vi "Instrument Sequence Loop.vi"(6 "Which Program?":T1, 8 "error in":errorcluster, 10 "Message Queues out":T15, 11 "Notifiers":T2) -> (0 "error out":errorcluster)   [LabVIEW 2014]
uses:
  support/Message Queue/All Message Queues.ctl
  support/Message Queue/Message Cluster.ctl
  support/Notifiers/Notifiers.ctl
  support/Message Handler Loop Notifiers.ctl
  Hardware Control/Parameter Analyzer/Parameter Analyzer Notifiers.ctl
  Hardware Control/Switching Matrix/Switching Matrix Notifiers.ctl
  Hardware Control/Stress Control/StressControl Notifiers.ctl
  Hardware Control/Spectrometer/Spectrometer Notifiers.ctl
  Hardware Control/Switches and Mirrors/SwitchesMirrors Notifiers.ctl
  Hardware Control/Camera/Camera Notifiers.ctl
  Hardware Control/XYZ Stage/XYZ Notifications.ctl
  Hardware Control/Autofocus/Autofocus Notifiers.ctl
  Measurements/Optoelectronic Measurement/Optoelectronic Notifiers.ctl
  Measurements/Save Data/SaveData Notifiers.ctl
  Measurements/Instrument Sequence/Instrument Sequence Notifiers.ctl
  Measurements/Instrument Sequence/Instrument Stequence - Which Program.ctl
  Measurements/Instrument Sequence/Instrument Sequence Function.ctl
  support/Message Queue/Message Queue.lvlib
panel:
  # "LICENSED MATERIALS – PROPERTY OF IBM\nCopyright IBM Corp. 2016,\nALL RIGHTS RESERVED"
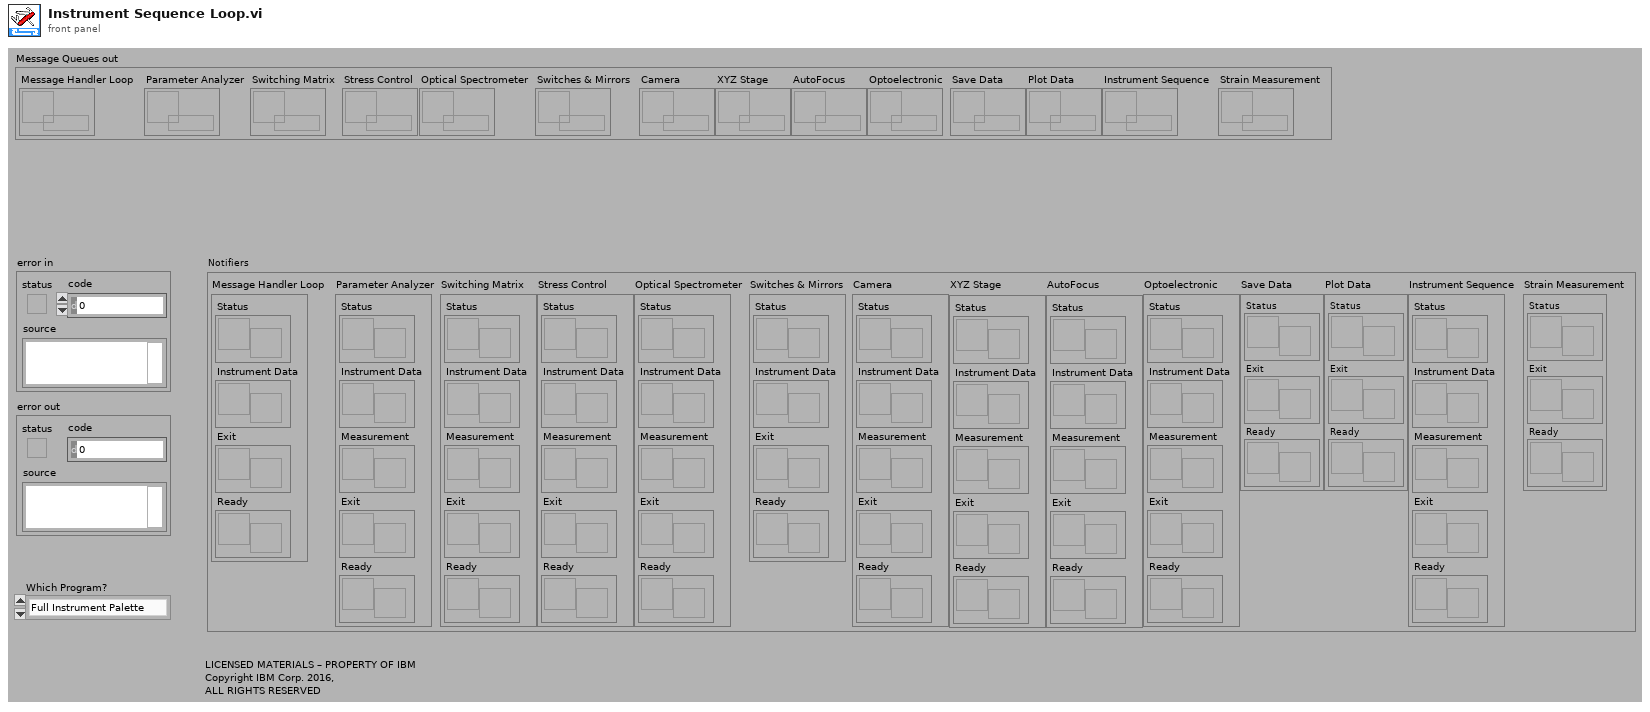
[diagram p1: front panel]
types:
  T1 = typedef "Instrument Stequence - Which Program.ctl" = enum16{"Full Instrument Palette", "Strain Electrical"}
  T2 = typedef "Notifiers.ctl" = cluster{"Message Handler Loop":T3, "Parameter Analyzer":T4, "Switching Matrix":T5, "Stress Control":T6, "Optical Spectrometer":T7, "Switches & Mirrors":T8, "Camera":T9, "XYZ Stage":T10, "AutoFocus":T11, "Optoelectronic":T12, "Save Data":T13, "Plot Data":T13, "Instrument Sequence":T14, "Strain Measurement":cluster{"Status":refnum<notifier>, "Exit":refnum<notifier>, "Ready":refnum<notifier>}}
  T3 = typedef "Message Handler Loop Notifiers.ctl" = cluster{"Status":refnum<notifier>, "Instrument Data":refnum<notifier>, "Exit":refnum<notifier>, "Ready":refnum<notifier>}
  T4 = typedef "Parameter Analyzer Notifiers.ctl" = cluster{"Status":refnum<notifier>, "Instrument Data":refnum<notifier>, "Measurement":refnum<notifier>, "Exit":refnum<notifier>, "Ready":refnum<notifier>}
  T5 = typedef "Switching Matrix Notifiers.ctl" = cluster{"Status":refnum<notifier>, "Instrument Data":refnum<notifier>, "Measurement":refnum<notifier>, "Exit":refnum<notifier>, "Ready":refnum<notifier>}
  T6 = typedef "StressControl Notifiers.ctl" = cluster{"Status":refnum<notifier>, "Instrument Data":refnum<notifier>, "Measurement":refnum<notifier>, "Exit":refnum<notifier>, "Ready":refnum<notifier>}
  T7 = typedef "Spectrometer Notifiers.ctl" = cluster{"Status":refnum<notifier>, "Instrument Data":refnum<notifier>, "Measurement":refnum<notifier>, "Exit":refnum<notifier>, "Ready":refnum<notifier>}
  T8 = typedef "SwitchesMirrors Notifiers.ctl" = cluster{"Status":refnum<notifier>, "Instrument Data":refnum<notifier>, "Exit":refnum<notifier>, "Ready":refnum<notifier>}
  T9 = typedef "Camera Notifiers.ctl" = cluster{"Status":refnum<notifier>, "Instrument Data":refnum<notifier>, "Measurement":refnum<notifier>, "Exit":refnum<notifier>, "Ready":refnum<notifier>}
  T10 = typedef "XYZ Notifications.ctl" = cluster{"Status":refnum<notifier>, "Instrument Data":refnum<notifier>, "Measurement":refnum<notifier>, "Exit":refnum<notifier>, "Ready":refnum<notifier>}
  T11 = typedef "Autofocus Notifiers.ctl" = cluster{"Status":refnum<notifier>, "Instrument Data":refnum<notifier>, "Measurement":refnum<notifier>, "Exit":refnum<notifier>, "Ready":refnum<notifier>}
  T12 = typedef "Optoelectronic Notifiers.ctl" = cluster{"Status":refnum<notifier>, "Instrument Data":refnum<notifier>, "Measurement":refnum<notifier>, "Exit":refnum<notifier>, "Ready":refnum<notifier>}
  T13 = typedef "SaveData Notifiers.ctl" = cluster{"Status":refnum<notifier>, "Exit":refnum<notifier>, "Ready":refnum<notifier>}
  T14 = typedef "Instrument Sequence Notifiers.ctl" = cluster{"Status":refnum<notifier>, "Instrument Data":refnum<notifier>, "Measurement":refnum<notifier>, "Exit":refnum<notifier>, "Ready":refnum<notifier>}
  T15 = typedef "Message Queue.lvlib/All Message Queues.ctl" = cluster{"Message Handler Loop":refnum<queue>, "Parameter Analyzer":refnum<queue>, "Switching Matrix":refnum<queue>, "Stress Control":refnum<queue>, "Optical Spectrometer":refnum<queue>, "Switches & Mirrors":refnum<queue>, "Camera":refnum<queue>, "XYZ Stage":refnum<queue>, "AutoFocus":refnum<queue>, "Optoelectronic":refnum<queue>, "Save Data":refnum<queue>, "Plot Data":refnum<queue>, "Instrument Sequence":refnum<queue>, "Strain Measurement":refnum<queue>}
  T16 = typedef "Instrument Sequence Data.ctl" = cluster{"Configuration":T17, "Refnums":T18}
  T17 = typedef "Instrument Sequence Config.ctl" = cluster{"Caller VI":enum16{"User", "Stress Measurement VI"}}
  T18 = typedef "Instrument Sequence Refnums.ctl" = cluster{"Instrument Steps":refnum<vi>, "Instruments Status":refnum<vi>, "Device ID":refnum<vi>, "Device Information":refnum<vi>, "Pause-Resume":refnum<vi>, "Plot":T19}
  T19 = typedef "Electrical Data Plot Refnums.ctl" = cluster{"Plot List":refnum<vi>, "Voltage Plot":refnum<vi>, "Current Plot":refnum<vi>, "IV Characteristic":refnum<vi>, "dI/dV-V Characteristic":refnum<vi>}
  T20 = typedef "Instrument Sequence Function.ctl" = enum16{"Update Refnums", "Get Instruments Status", "Initialize Dialog", "Get Autofocus Status", "Add Step", "Remove Step", "Clear Sequence", "Load Sequence", "Save Sequence", "Measure Sequence", "Reset Sequence", "Start Sequence", "Start Sequence for Strain Measurement", "Stop Sequence", "Pause Sequence", "Update Sequence Status", "Choose What Next", "Update Workspace Data", "Save Measured Sequence", "Configure Parameter Analyzer", "Perform Electrical Measurement", "Configure Switching Matrix", "Configure Optical Spectrometer", "Focus", "Perform Optical Measurement", "Perform Optoelectronic Measurement", "Declare Completion"}
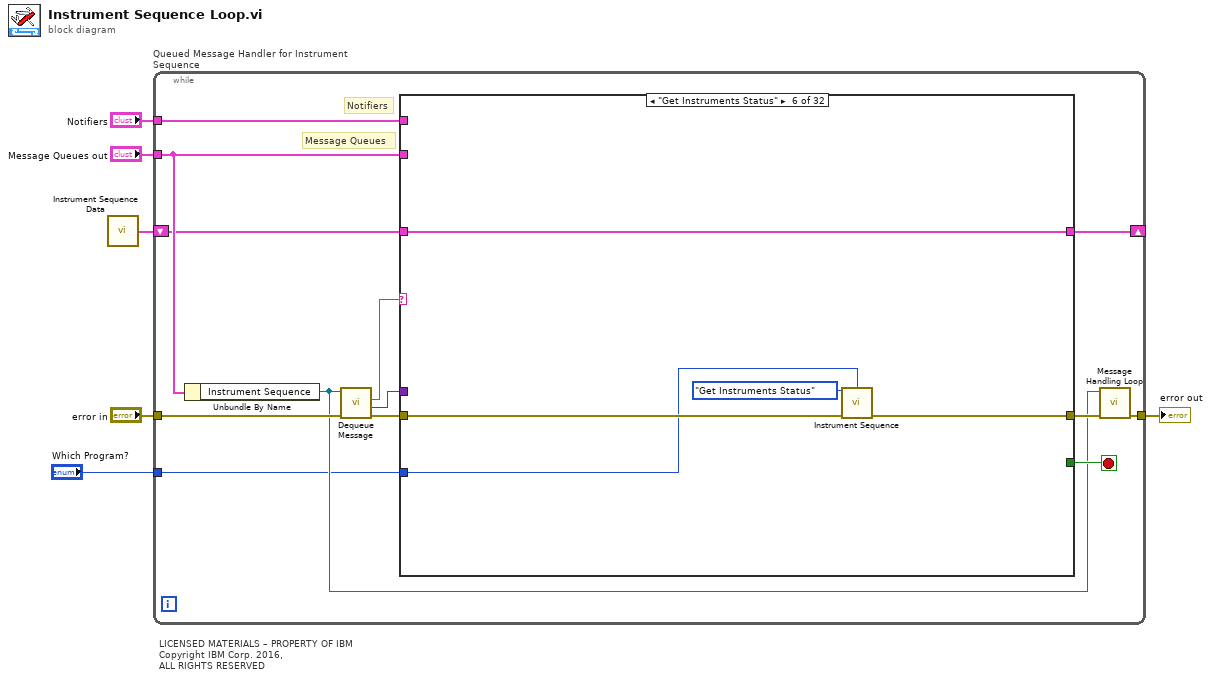
[diagram p0: block diagram]
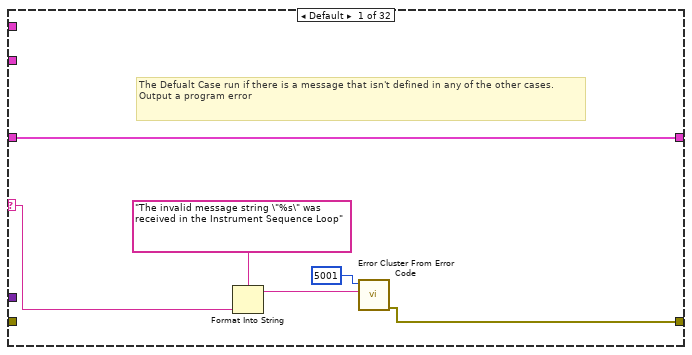
[diagram p2: hidden frame]
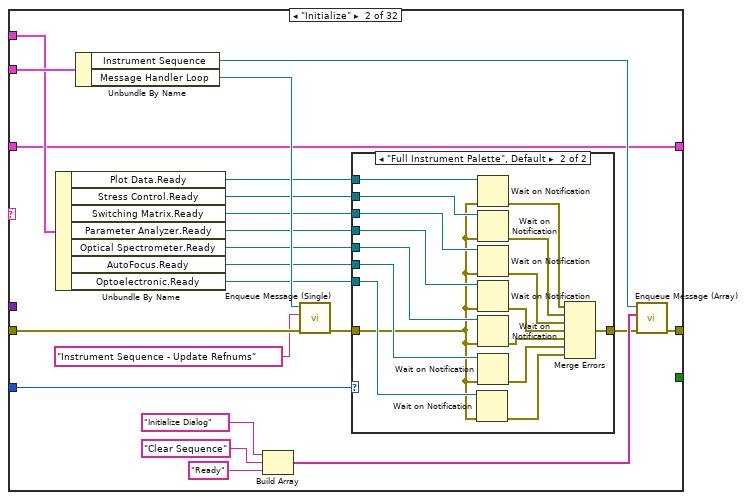
[diagram p3: hidden frame]
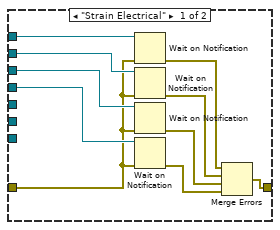
[diagram p4: hidden frame]
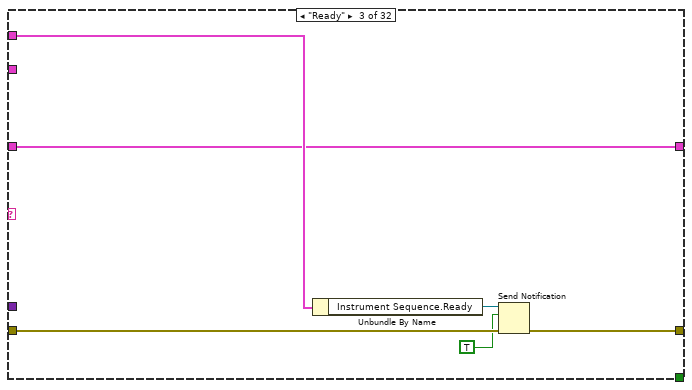
[diagram p5: hidden frame]
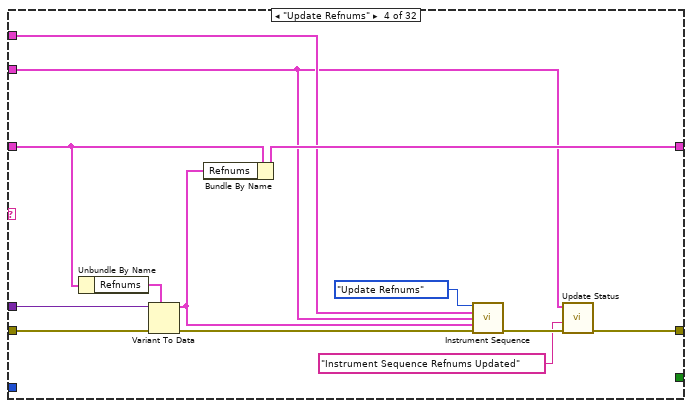
[diagram p6: hidden frame]
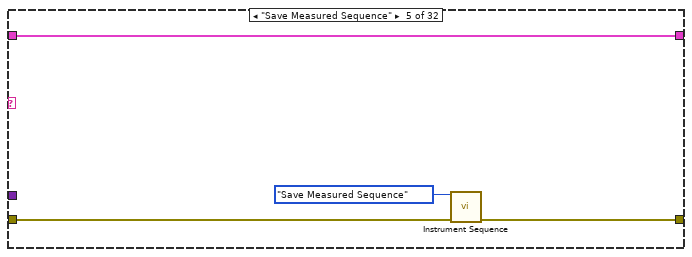
[diagram p7: hidden frame]
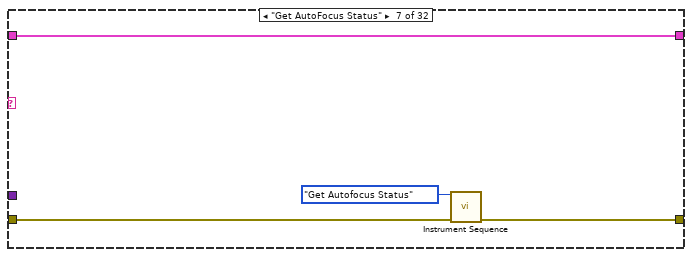
[diagram p8: hidden frame]
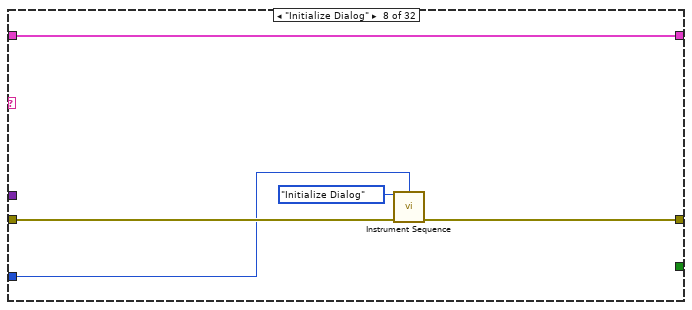
[diagram p9: hidden frame]
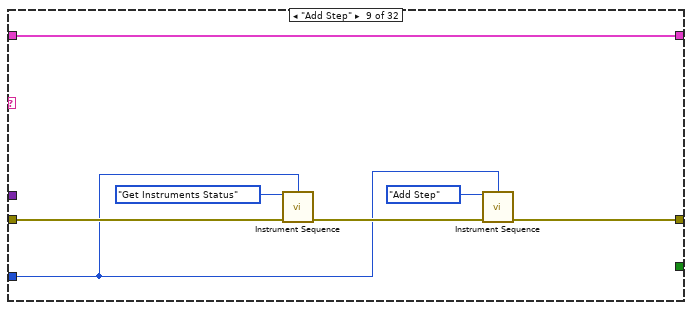
[diagram p10: hidden frame]
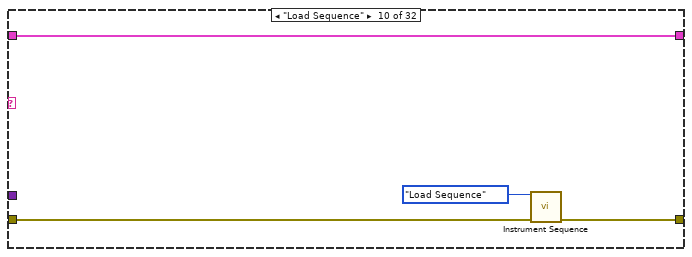
[diagram p11: hidden frame]
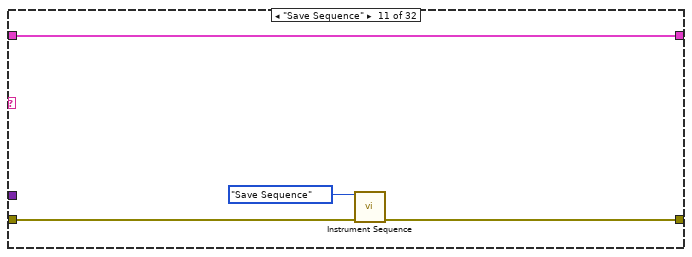
[diagram p12: hidden frame]
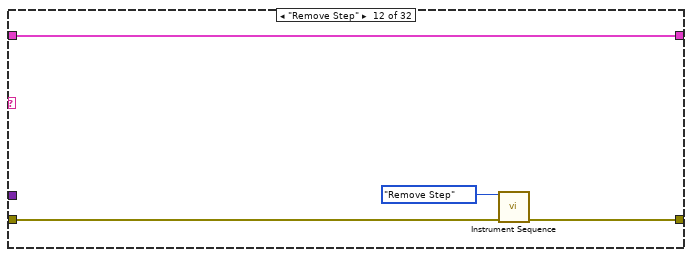
[diagram p13: hidden frame]
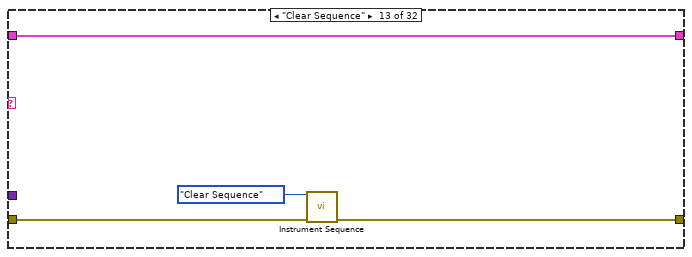
[diagram p14: hidden frame]
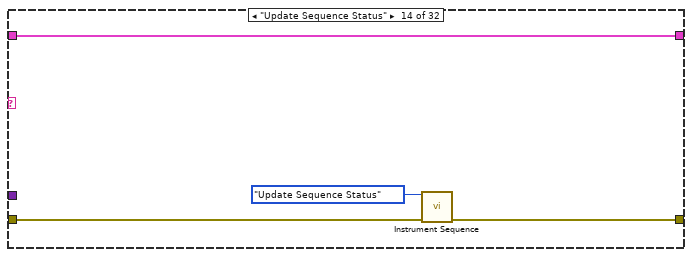
[diagram p15: hidden frame]
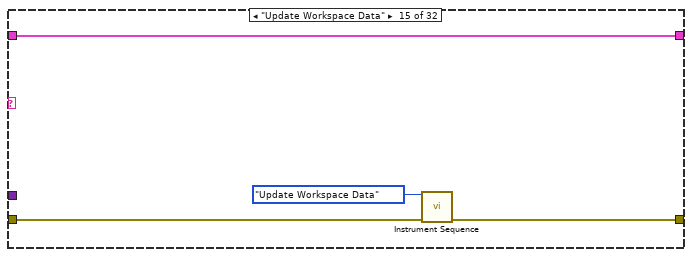
[diagram p16: hidden frame]
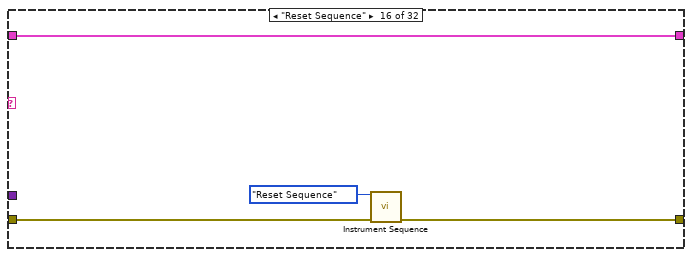
[diagram p17: hidden frame]
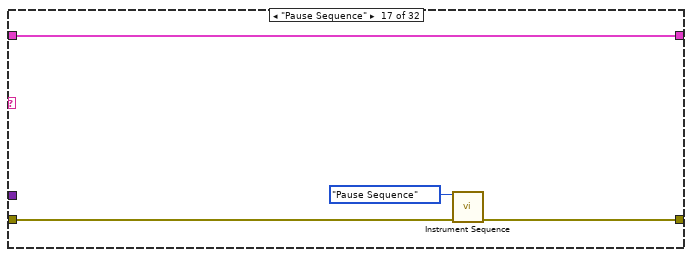
[diagram p18: hidden frame]
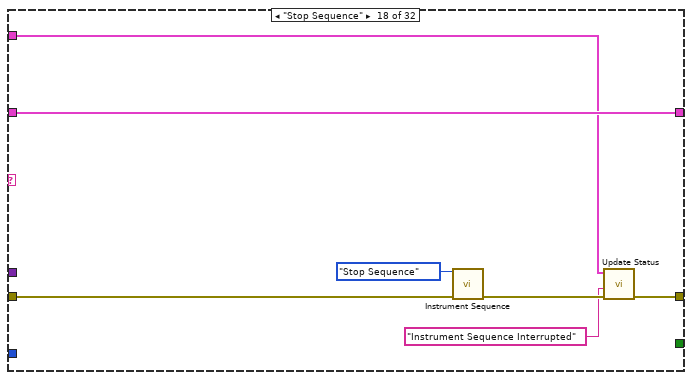
[diagram p19: hidden frame]
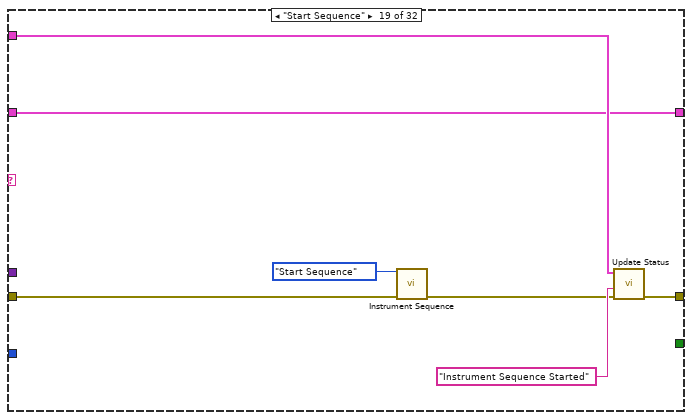
[diagram p20: hidden frame]
diagram:
  # "LICENSED MATERIALS – PROPERTY OF IBM\nCopyright IBM Corp. 2016,\nALL RIGHTS RESERVED"
  n1 = call "Instrument Sequence Data.vi"() -> ("Instrument Sequence Data"=w2:T16)
  n2 = while "Queued Message Handler for Instrument Sequence" {
    tunnel: "error in" -> [w19]
    tunnel: [w11] -> w3
    tunnel: "Message Queues out" -> [w15]
    tunnel: "Notifiers" -> [w14]
    shift-right: [w8] -> _
    shift-left: w2 -> [w9]
    tunnel: "Which Program?" -> [w7]
    stop <- w13 stop-if-true
    # "Notifiers"
    # "Message Queues"
    n3 = Unbundle By Name(w15) -> ("Instrument Sequence"=w10:refnum<queue>)
    n4 = call "Dequeue Message.vi"("error in (no error)"=w19, "Message Queue"=w10) -> ("error out"=w18:errorcluster, "Message Data"=w16:variant, "Message"=w17:string)  [unwired: 7 out]
    n5 = case shown="\"Get Instruments Status\"" w17 {
      selector: w17 -> [w22 _ _ _ _ _ _ _ _ _ _ _ _ _ _ _ _ _ _ _ _ _ _ _ _ _ _ _ _ _ _ _]
      tunnel: w18 -> [_ w45 w76 w91 w95 w99 w103 w109 w113 w118 w122 w126 w131 w136 w140 w142 w147 w154 w158 w169 w175 w182 w190 w199 w205 w210 w214 w217 w221 w225 w236 w251]
      tunnel: [w21 w37 w79 w90 w93 w98 w102 w108 w115 w119 w124 w127 w130 w134 w138 w144 w146 w152 w162 w170 w173 w183 w188 w201 w204 w209 w213 w216 w220 w224 w231 w244] -> w12
      tunnel: w16 -> [_ _ _ w92 _ _ _ _ _ _ _ _ _ _ _ _ _ _ _ w167 _ w179 _ w197 w202 w207 _ _ _ _ w229 _]
      tunnel: w15 -> [_ w47 _ w84 _ _ _ _ _ _ _ _ _ _ _ _ _ w151 w161 _ _ _ w186 _ _ _ _ _ _ _ w237 w254]
      tunnel: w14 -> [_ w46 w77 w85 _ _ _ _ _ _ _ _ _ _ _ _ _ _ _ _ _ _ _ _ _ _ _ _ _ _ _ w246]
      tunnel: [_ _ _ _ _ _ _ _ _ _ _ _ _ _ _ _ _ _ _ _ _ _ _ _ _ _ _ _ _ _ _ TRUE ("Priority Message? (F)")] -> w13
      tunnel: w9 -> [w20 w33 w74 w88 w96 w101 w105 w110 w116 w120 w123 w128 w132 w137 w141 w143 w149 w156 w159 w166 w174 w181 w189 w198 w206 w211 w215 w219 w223 w227 w228 w252]
      tunnel: [w20 w33 w74 w89 w96 w101 w105 w110 w116 w120 w123 w128 w132 w137 w141 w143 w149 w156 w159 w171 w174 w178 w189 w198 w206 w211 w215 w219 w223 w227 w228 w252] -> w8
      tunnel: w7 -> [_ w27 _ _ _ w97 _ w106 w111 _ _ _ _ _ _ _ _ _ _ _ _ _ _ _ _ _ _ _ _ _ _ _]
      frame Default {
        # "The Defualt Case run if there is a message that isn't defined in any of the other cases.\nOutput a program error"
        n6 = Format Into String(format string="The invalid message string \"%s\" was  received in the Instrument Sequence Loop", w22) -> (resulting string=w24:string)  [unwired: 2 in, 1 out]
        n7 = call <vilib>:"Error Cluster From Error Code.vi"("error message (\"\")"=w24, "error code (0)"=5001) -> ("error out"=w21:errorcluster)  [unwired: 2 in, 5 out]
      }
      frame "Initialize" {
        n8 = Unbundle By Name(w46) -> ("Plot Data.Ready"=w28:refnum<notifier>, "Stress Control.Ready"=w40:refnum<notifier>, "Switching Matrix.Ready"=w42:refnum<notifier>, "Parameter Analyzer.Ready"=w41:refnum<notifier>, "Optical Spectrometer.Ready"=w31:refnum<notifier>, "AutoFocus.Ready"=w30:refnum<notifier>, "Optoelectronic.Ready"=w26:refnum<notifier>)
        n9 = Unbundle By Name(w47) -> ("Instrument Sequence"=w39:refnum<queue>, "Message Handler Loop"=w43:refnum<queue>)
        n10 = Build Array("Initialize Dialog" ("Message"), "Clear Sequence" ("Message"), "Ready" ("Message")) -> (w38:string[])
        n11 = call "Enqueue Message (Single).vi"("error in (no error)"=w45, "Message"="Instrument Sequence - Update Refnums", "Message Queue"=w43) -> ("error out"=w29:errorcluster)  [unwired: 1 in, 7 out]
        n12 = case shown="\"Full Instrument Palette\", Default" w27 {
          tunnel: w42 -> [w57 w73]
          tunnel: w41 -> [w56 w72]
          tunnel: w40 -> [w54 w70]
          tunnel: [w50 w66] -> w32
          tunnel: w31 -> [_ w64]
          tunnel: w30 -> [_ w63]
          tunnel: w29 -> [w49 w59]
          tunnel: w28 -> [w48 w61]
          tunnel: w26 -> [_ w60]
          frame "Strain Electrical" {
            n13 = Wait on Notification(notifier=w48, error in (no error)=w49) -> (error out=w51:errorcluster)  [unwired: 5 out]
            n14 = Wait on Notification(notifier=w54, error in (no error)=w49) -> (error out=w52:errorcluster)  [unwired: 5 out]
            n15 = Wait on Notification(notifier=w57, error in (no error)=w49) -> (error out=w53:errorcluster)  [unwired: 5 out]
            n16 = Wait on Notification(notifier=w56, error in (no error)=w49) -> (error out=w55:errorcluster)  [unwired: 5 out]
            n17 = Merge Errors(w51, w52, w53, w55) -> (w50:errorcluster)
          }
          frame "Full Instrument Palette", Default {
            n18 = Wait on Notification(notifier=w60, error in (no error)=w59) -> (error out=w58:errorcluster)  [unwired: 5 out]
            n19 = Wait on Notification(notifier=w61, error in (no error)=w59) -> (error out=w67:errorcluster)  [unwired: 5 out]
            n20 = Wait on Notification(notifier=w70, error in (no error)=w59) -> (error out=w68:errorcluster)  [unwired: 5 out]
            n21 = Wait on Notification(notifier=w73, error in (no error)=w59) -> (error out=w69:errorcluster)  [unwired: 5 out]
            n22 = Wait on Notification(notifier=w72, error in (no error)=w59) -> (error out=w71:errorcluster)  [unwired: 5 out]
            n23 = Wait on Notification(notifier=w64, error in (no error)=w59) -> (error out=w65:errorcluster)  [unwired: 5 out]
            n24 = Wait on Notification(notifier=w63, error in (no error)=w59) -> (error out=w62:errorcluster)  [unwired: 5 out]
            n25 = Merge Errors(w67, w68, w69, w71, w65, w62, w58) -> (w66:errorcluster)
          }
        }
        n26 = call "Enqueue Message (Array).vi"("error in (no error)"=w32, "Message Array"=w38, "Message Queue"=w39) -> ("error out"=w37:errorcluster)  [unwired: 1 in, 7 out]
      }
      frame "Ready" {
        n27 = Unbundle By Name(w77) -> ("Instrument Sequence.Ready"=w78:refnum<notifier>)
        n28 = Send Notification(notification=TRUE, notifier=w78, error in (no error)=w76) -> (error out=w79:errorcluster)  [unwired: 1 out]
      }
      frame "Update Refnums" {
        n29 = Unbundle By Name(w88) -> ("Refnums"=w87:T18)
        n30 = Variant To Data(error in=w91, type=w87, Variant=w92) -> (data=w81:T18, error out=w83:errorcluster)
        n31 = Bundle By Name(cluster=w88, "Refnums"=w81) -> (w89:T16)
        n32 = call "Instrument Sequence.vi"("Function"=Instrument_Sequence_Function."Update Refnums", "Notifiers"=w85, "Message Queues"=w84, "Refnums"=w81, "error in (no error)"=w83) -> ("error out"=w82:errorcluster)  [unwired: 3 in, 7 out]
        n33 = call "Update Status.vi"("error in"=w82, "String"="Instrument Sequence Refnums Updated", "Message Queues out"=w84) -> ("error out"=w90:errorcluster)  [unwired: 8 out]
      }
      frame "Save Measured Sequence" {
        n34 = call "Instrument Sequence.vi"("Function"=Instrument_Sequence_Function."Save Measured Sequence", "error in (no error)"=w95) -> ("error out"=w93:errorcluster)  [unwired: 6 in, 7 out]
      }
      frame "Get Instruments Status" {
        n35 = call "Instrument Sequence.vi"("Function"=Instrument_Sequence_Function."Get Instruments Status", "Which Program?"=w97, "error in (no error)"=w99) -> ("error out"=w98:errorcluster)  [unwired: 5 in, 7 out]
      }
      frame "Get AutoFocus Status" {
        n36 = call "Instrument Sequence.vi"("Function"=Instrument_Sequence_Function."Get Autofocus Status", "error in (no error)"=w103) -> ("error out"=w102:errorcluster)  [unwired: 6 in, 7 out]
      }
      frame "Initialize Dialog" {
        n37 = call "Instrument Sequence.vi"("Function"=Instrument_Sequence_Function."Initialize Dialog", "Which Program?"=w106, "error in (no error)"=w109) -> ("error out"=w108:errorcluster)  [unwired: 5 in, 7 out]
      }
      frame "Add Step" {
        n38 = call "Instrument Sequence.vi"("Function"=Instrument_Sequence_Function."Get Instruments Status", "Which Program?"=w111, "error in (no error)"=w113) -> ("error out"=w112:errorcluster)  [unwired: 5 in, 7 out]
        n39 = call "Instrument Sequence.vi"("Function"=Instrument_Sequence_Function."Add Step", "Which Program?"=w111, "error in (no error)"=w112) -> ("error out"=w115:errorcluster)  [unwired: 5 in, 7 out]
      }
      frame "Load Sequence" {
        n40 = call "Instrument Sequence.vi"("Function"=Instrument_Sequence_Function."Load Sequence", "error in (no error)"=w118) -> ("error out"=w119:errorcluster)  [unwired: 6 in, 7 out]
      }
      frame "Save Sequence" {
        n41 = call "Instrument Sequence.vi"("Function"=Instrument_Sequence_Function."Save Sequence", "error in (no error)"=w122) -> ("error out"=w124:errorcluster)  [unwired: 6 in, 7 out]
      }
      frame "Remove Step" {
        n42 = call "Instrument Sequence.vi"("Function"=Instrument_Sequence_Function."Remove Step", "error in (no error)"=w126) -> ("error out"=w127:errorcluster)  [unwired: 6 in, 7 out]
      }
      frame "Clear Sequence" {
        n43 = call "Instrument Sequence.vi"("Function"=Instrument_Sequence_Function."Clear Sequence", "error in (no error)"=w131) -> ("error out"=w130:errorcluster)  [unwired: 6 in, 7 out]
      }
      frame "Update Sequence Status" {
        n44 = call "Instrument Sequence.vi"("Function"=Instrument_Sequence_Function."Update Sequence Status", "error in (no error)"=w136) -> ("error out"=w134:errorcluster)  [unwired: 6 in, 7 out]
      }
      frame "Update Workspace Data" {
        n45 = call "Instrument Sequence.vi"("Function"=Instrument_Sequence_Function."Update Workspace Data", "error in (no error)"=w140) -> ("error out"=w138:errorcluster)  [unwired: 6 in, 7 out]
      }
      frame "Reset Sequence" {
        n46 = call "Instrument Sequence.vi"("Function"=Instrument_Sequence_Function."Reset Sequence", "error in (no error)"=w142) -> ("error out"=w144:errorcluster)  [unwired: 6 in, 7 out]
      }
      frame "Pause Sequence" {
        n47 = call "Instrument Sequence.vi"("Function"=Instrument_Sequence_Function."Pause Sequence", "error in (no error)"=w147) -> ("error out"=w146:errorcluster)  [unwired: 6 in, 7 out]
      }
      frame "Stop Sequence" {
        n48 = call "Instrument Sequence.vi"("Function"=Instrument_Sequence_Function."Stop Sequence", "error in (no error)"=w154) -> ("error out"=w153:errorcluster)  [unwired: 6 in, 7 out]
        n49 = call "Update Status.vi"("error in"=w153, "String"="Instrument Sequence Interrupted", "Message Queues out"=w151) -> ("error out"=w152:errorcluster)  [unwired: 8 out]
      }
      frame "Start Sequence" {
        n50 = call "Instrument Sequence.vi"("Function"=Instrument_Sequence_Function."Start Sequence", "error in (no error)"=w158) -> ("error out"=w157:errorcluster)  [unwired: 6 in, 7 out]
        n51 = call "Update Status.vi"("error in"=w157, "String"="Instrument Sequence Started", "Message Queues out"=w161) -> ("error out"=w162:errorcluster)  [unwired: 8 out]
      }
      frame "Measure Sequence" {
        n52 = Unbundle By Name(w166) -> ("Configuration.Caller VI"=w165:enum16{"User", "Stress Measurement VI"})
        n53 = Variant To Data(error in=w169, type=w165, Variant=w167) -> (data=w164:enum16{"User", "Stress Measurement VI"}, error out=w168:errorcluster)
        n54 = call "Instrument Sequence.vi"("Function"=Instrument_Sequence_Function."Measure Sequence", "Caller VI"=w164, "error in (no error)"=w168) -> ("error out"=w170:errorcluster)  [unwired: 5 in, 7 out]
        n55 = Bundle By Name(cluster=w166, "Configuration.Caller VI"=w164) -> (w171:T16)
      }
      frame "Start Sequence for Strain Measurement" {
        n56 = call "Instrument Sequence.vi"("Function"=Instrument_Sequence_Function."Start Sequence for Strain Measurement", "error in (no error)"=w175) -> ("error out"=w173:errorcluster)  [unwired: 6 in, 7 out]
      }
      frame "Choose What Next" {
        n57 = Unbundle By Name(w181) -> ("Configuration.Caller VI"=w177:enum16{"User", "Stress Measurement VI"})
        n58 = Variant To Data(error in=w182, type=w177, Variant=w179) -> (error out=w180:errorcluster)  [unwired: 1 out]
        n59 = call "Instrument Sequence.vi"("Function"=Instrument_Sequence_Function."Choose What Next", "Caller VI"=w177, "error in (no error)"=w180) -> ("error out"=w183:errorcluster)  [unwired: 5 in, 7 out]
        n60 = Bundle By Name(cluster=w181, "Configuration.Caller VI"=w177) -> (w178:T16)
      }
      frame "Declare Completion" {
        n61 = Unbundle By Name(w189) -> ("Configuration.Caller VI"=w185:enum16{"User", "Stress Measurement VI"})
        n62 = call "Instrument Sequence.vi"("Function"=Instrument_Sequence_Function."Declare Completion", "Caller VI"=w185, "error in (no error)"=w190) -> ("error out"=w187:errorcluster)  [unwired: 5 in, 7 out]
        n63 = case shown="\"User\", Default" w185 {
          tunnel: [w195 w196] -> w188
          tunnel: w187 -> [w194 w196]
          tunnel: w186 -> [w193 _]
          frame "User", Default {
            n64 = call "Update Status.vi"("error in"=w194, "String"="Instrument Sequence Completed", "Message Queues out"=w193) -> ("error out"=w195:errorcluster)  [unwired: 8 out]
          }
          frame "Stress Measurement VI" {
          }
        }
      }
      frame "Configure Parameter Analyzer" {
        n65 = call "Instrument Sequence.vi"("Function"=Instrument_Sequence_Function."Configure Parameter Analyzer", "error in (no error)"=w199, "Configuration"=w197) -> ("error out"=w201:errorcluster)  [unwired: 5 in, 7 out]
      }
      frame "Configure Switching Matrix" {
        n66 = call "Instrument Sequence.vi"("Function"=Instrument_Sequence_Function."Configure Switching Matrix", "error in (no error)"=w205, "Configuration"=w202) -> ("error out"=w204:errorcluster)  [unwired: 5 in, 7 out]
      }
      frame "Configure Optical Spectrometer" {
        n67 = call "Instrument Sequence.vi"("Function"=Instrument_Sequence_Function."Configure Optical Spectrometer", "error in (no error)"=w210, "Configuration"=w207) -> ("error out"=w209:errorcluster)  [unwired: 5 in, 7 out]
      }
      frame "Focus" {
        n68 = call "Instrument Sequence.vi"("Function"=Instrument_Sequence_Function."Focus", "error in (no error)"=w214) -> ("error out"=w213:errorcluster)  [unwired: 6 in, 7 out]
      }
      frame "Perform Electrical Measurement" {
        n69 = call "Instrument Sequence.vi"("Function"=Instrument_Sequence_Function."Perform Electrical Measurement", "error in (no error)"=w217) -> ("error out"=w216:errorcluster)  [unwired: 6 in, 7 out]
      }
      frame "Perform Optical Measurement" {
        n70 = call "Instrument Sequence.vi"("Function"=Instrument_Sequence_Function."Perform Optical Measurement", "error in (no error)"=w221) -> ("error out"=w220:errorcluster)  [unwired: 6 in, 7 out]
      }
      frame "Perform Optoelectronic Measurement" {
        n71 = call "Instrument Sequence.vi"("Function"=Instrument_Sequence_Function."Perform Optoelectronic Measurement", "error in (no error)"=w225) -> ("error out"=w224:errorcluster)  [unwired: 6 in, 7 out]
      }
      frame "Error" {
        # "Clear Errors to avoid getting stuck \nin repeating this case"
        # "Add here Cases that are handled \nalready by the Message Handler Loop"
        n72 = Variant To Data(error in=w236, type=errorcluster {"status"=FALSE, "code"=0, "source"=""} ("error out"), Variant=w229) -> (data=w235:errorcluster, error out=w234:errorcluster)
        n73 = Merge Errors(w235, w234) -> (w233:errorcluster)
        n74 = Unbundle By Name(w237) -> ("Message Handler Loop"=w239:refnum<queue>)
        n75 = Unbundle By Name(w233) -> ("code"=w230:i32)
        n76 = case shown="Default" w230 {
          tunnel: w239 -> [w243]
          tunnel: w233 -> [w241]
          tunnel: [w240] -> w232
          frame Default {
            n77 = call "Enqueue Message (Single).vi"("Message Data"=w241, "Message"="Error", "Message Queue"=w243) -> ("error out"=w240:errorcluster)  [unwired: 1 in, 7 out]
          }
        }
        n78 = call <vilib>:"Clear Errors.vi"("error in (no error)"=w232) -> ("error out"=w231:errorcluster)  [unwired: 1 in, 5 out]
      }
      frame "Exit" {
        w249 = TRUE ("Priority Message? (F)")
        # "Stip the VI"
        n79 = Unbundle By Name(w254) -> ("Instrument Sequence"=w255:refnum<queue>)
        n80 = Release Queue(queue=w255, error in (no error)=w251) -> (error out=w245:errorcluster)  [unwired: 3 out]
        n81 = Unbundle By Name(w246) -> ("Instrument Sequence.Exit"=w250:refnum<notifier>, "Instrument Sequence.Ready"=w247:refnum<notifier>)
        n82 = Send Notification(notification=w249, notifier=w247, error in (no error)=w245) -> (error out=w248:errorcluster)  [unwired: 1 out]
        n83 = Send Notification(notification=w249, notifier=w250, error in (no error)=w248) -> (error out=w244:errorcluster)  [unwired: 1 out]
      }
    }
    n84 = call "Message Handling Loop.vi"("error in (no error)"=w12, "Message Queue"=w10) -> ("dup error in"=w11:errorcluster)  [unwired: 9 out]
  }
  "error out" <- w3
